vi "Text List to Array.vi"(1 "delimiter (;)":string=";", 3 "text list":string) -> (0 "array":dbl[](array[numeric]))   [LabVIEW 2020]
doc: "Converts a semicolon delimited text list into an array of doubles."
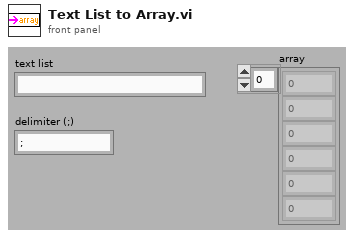
[diagram p1: front panel]
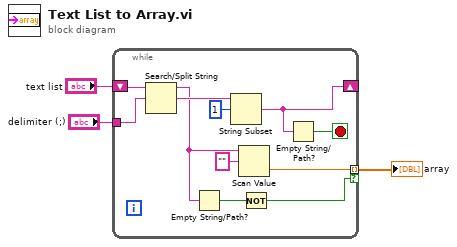
[diagram p0: block diagram]
diagram:
  n1 = while {
    shift-right: [w8] -> _
    shift-left: "text list" -> [w14]
    tunnel: "delimiter (;)" -> [w12]
    tunnel: [w5] -> w1 mode=indexing if=w10
    stop <- w7 stop-if-true
    n2 = Search/Split String(string=w14, search string/char (-)=w12) -> (substring before match=w6:string, match + rest of string=w13:string)  [unwired: 1 in, 1 out]
    n3 = Empty String/Path?(string/path=w6) -> (empty?=w11:bool)
    n4 = String Subset(string=w13, offset (0)=1) -> (substring=w8:string)  [unwired: 1 in]
    n5 = Scan Value(string=w6, format string="") -> (value=w5:dbl)  [unwired: 1 in, 1 out]
    n6 = Not(x=w11) -> (.not. x?=w10:bool)
    n7 = Empty String/Path?(string/path=w8) -> (empty?=w7:bool)
  }
  "array" <- w1
